vi "Serial_ClearBuffer.vi"(3 "error in (no error)":errorcluster) -> (0 "error out":errorcluster, 1 "read data":u8[](array[numeric]))   [LabVIEW 2009, in "Serial.lvlib"]
doc: "Clears all the data from Serial port buffer."
uses:
  Serial.lvlib
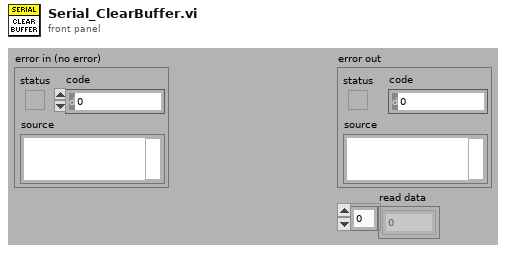
[diagram p1: front panel]
types:
  T1 = typedef "Semaphore RefNum" = refnum<k1>
  T2 = cluster{"VISA resource name":refnum<visa-resource-name>, "Semaphore":T1}
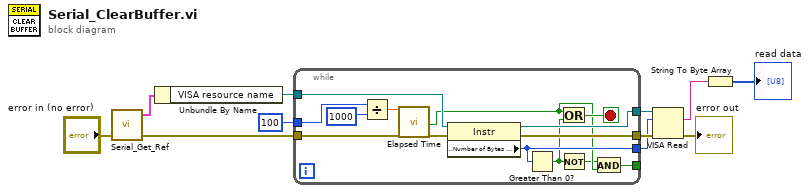
[diagram p0: block diagram]
diagram:
  n1 = call "Serial_Get_Ref.vi"("error in (no error)"="error in (no error)") -> ("error out"=w6:errorcluster, "Serial Ref"=w10:T2)  [unwired: 3 in]
  n2 = Unbundle By Name(w10) -> ("VISA resource name"=w8:refnum<visa-resource-name>)
  n3 = while {
    tunnel: u32 100 ("timeoutMs") -> [w18]
    tunnel: w6 -> [w20]
    tunnel: [w25] -> w4
    tunnel: [w23] -> w3
    tunnel: [w22] -> w5
    tunnel: w8 -> [w21]
    tunnel: [w15] -> _
    stop <- w24 stop-if-true
    n4 = Divide(x=w18, y=u32 1000) -> (x/y=w16:dbl)
    n5 = call "Elapsed Time"("Time Target (s)"=w16, "error in (no error)"=w20) -> ("Time has Elapsed"=w14:bool, "error out"=w19:errorcluster)  [unwired: 10 in, 6 out]
    n6 = property class="Instr"(reference=w21, error in=w19) -> (reference out=w22:refnum<visa-resource-name>, error out=w25:errorcluster, "Serial Settings:Number of Bytes at Serial Port"=w23:u32)
    n7 = Greater Than 0?(x=w23) -> (x > 0?=w12:bool)
    n8 = Or(x=w14, y=w12) -> (x .or. y?=w24:bool)
    n9 = Not(x=w12) -> (.not. x?=w13:bool)
    n10 = And(x=w13, y=w14) -> (x .and. y?=w15:bool)
  }
  n11 = VISA Read(VISA resource name=w5, byte count=w3, error in (no error)=w4) -> (read buffer=w2:string, error out=→"error out":errorcluster)  [unwired: 2 out]
  n12 = String To Byte Array(string=w2) -> (unsigned byte array=→"read data":u8[])
